vi "selectorenum.vi"(9 "Enum entrada":T2(ring), 10 "Orden":T1(array[ring]), 11 "arreglo opciones":bool[](array[boolean])) -> (2 "enum salida":T2(ring))   [LabVIEW 2016]
doc: "Este subVI funciona para seleccionar el estado que se va a ejecutar de acuerdo a el orden establecido por el usuario y a qué dispositivos definió para que se utilizaran.\n\nSus entradas son : \nEl arreglo orden que define el orden en el que se ejecutarán los dispositivos.\n\nEl arreglo opciones, que indica cuáles aparatos se utilizarán durante la medición.\n\nEl elemento que se supone debe de seguir en la secuencia\n\nComo salida es el elemento que continúa en la ejecución del programa."
panel:
  out "x = y?":bool
  out "index of element":i32
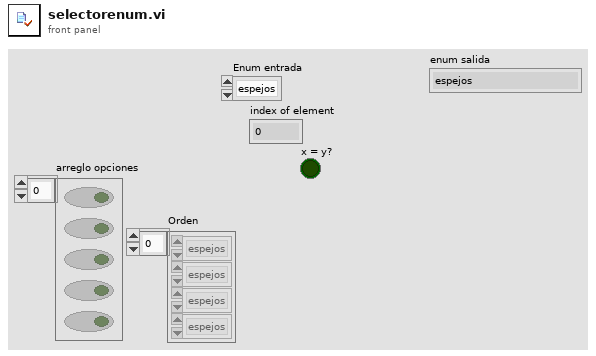
[diagram p1: front panel]
types:
  T1 = enum16{"espejos", "polarizador", "voltaje", "potenciometro y lockin", "CCD"}[]
  T2 = enum16{"espejos", "polarizador", "voltaje", "potenciometro y lockin", "CCD"}
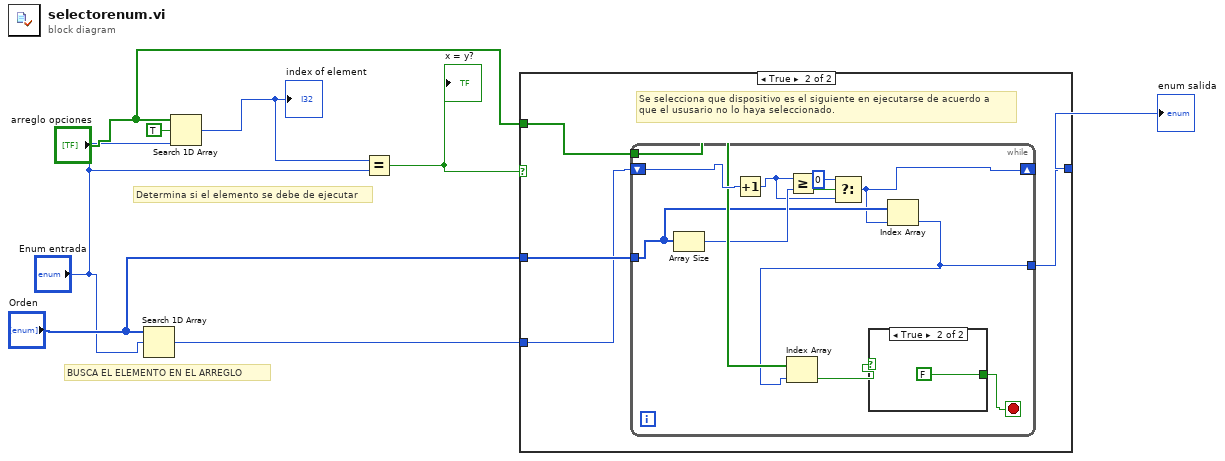
[diagram p0: block diagram]
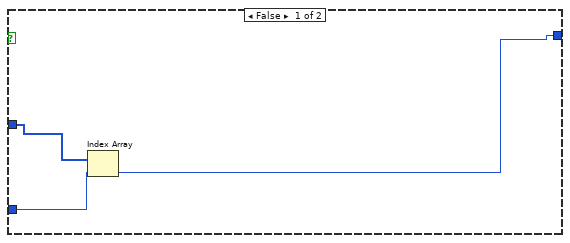
[diagram p2: hidden frame]
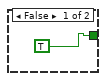
[diagram p3: hidden frame]
diagram:
  # "Determina si el elemento se debe de ejecutar"
  # "BUSCA EL ELEMENTO EN EL ARREGLO"
  n1 = Search 1D Array(1D array="Orden", element="Enum entrada") -> (index of element=w1:i32)  [unwired: 1 in]
  n2 = Search 1D Array(1D array="arreglo opciones", element=TRUE, start index (0)="Enum entrada") -> (index of element=w6:i32)
  "index of element" <- w6
  n3 = Equal?(x=w6, y="Enum entrada") -> (x = y?=w7:bool)
  "x = y?" <- w7
  n4 = case shown="True" w7 {
    tunnel: [w9 w12] -> w4
    tunnel: "arreglo opciones" -> [_ w15]
    tunnel: "Orden" -> [w11 w14]
    tunnel: w1 -> [w10 w13]
    frame False {
      n5 = Index Array(array=w11, index=w10) -> (element=w9:T2)
    }
    frame True {
      # "Se selecciona que dispositivo es el siguiente en ejecutarse de acuerdo a \nque el ususario no lo haya seleccionado."
      n6 = while {
        tunnel: w15 -> [w25]
        shift-right: [w16] -> _
        shift-left: w13 -> [w26]
        tunnel: w14 -> [w19]
        tunnel: [w18] -> w12
        stop <- w23 stop-if-true
        n7 = Array Size(array=w19) -> (size(s)=w22:i32)
        n8 = Increment(x=w26) -> (x+1=w17:i32)
        n9 = Greater Or Equal?(x=w17, y=w22) -> (x >= y?=w21:bool)
        n10 = Select(t=0, s=w21, f=w17) -> (s? t:f=w16:i32)
        n11 = Index Array(array=w19, index=w16) -> (element=w18:T2)
        n12 = Index Array(array=w25, index=w18) -> (element=w24:bool)
        n13 = case shown="True" w24 {
          tunnel: [TRUE FALSE] -> w23
          frame False {
          }
          frame True {
          }
        }
      }
    }
  }
  "enum salida" <- w4
